vi "globalAvion.vi"() -> ()   [LabVIEW 2014]
panel:
  out "Precision":dbl
  out "DatosValidos":dbl
  out "AvionVelocidad":dbl
  out "AvionAltitud":dbl
  out "AvionLongitud":dbl
  out "AvionLatitud":dbl
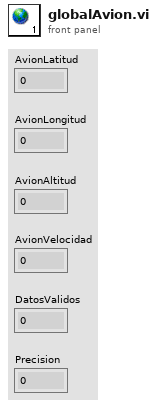
[diagram p1: front panel]
diagram:
